vi "CreateItemsString.vi"(11 "Items":string[](array[string])=["C1", "C2", "C3"]) -> (1 "Items for SELECT":string, 2 "Items for INSERT":string, 3 "Items for CREATE":string)   [LabVIEW 2015, in "DBToolkit.lvlib"]
uses:
  DBToolkit.lvlib
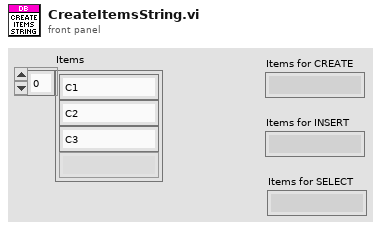
[diagram p1: front panel]
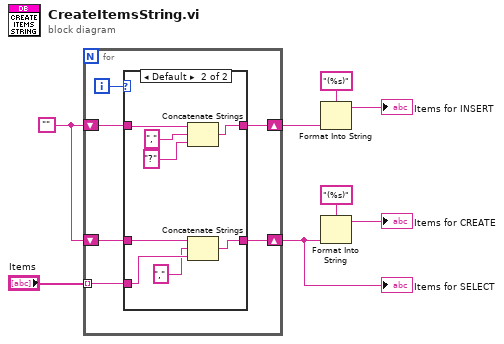
[diagram p0: block diagram]
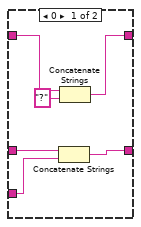
[diagram p2: hidden frame]
diagram:
  w7 = ""
  n1 = for {
    shift-right: [w11] -> w1
    shift-left: w7 -> [w13]
    tunnel: "Items" -> [w12] mode=indexing
    shift-right: [w9] -> w5
    shift-left: w7 -> [w10]
    i -> [w14]
    n2 = case shown="Default" w14 {
      tunnel: w13 -> [w20 w26]
      tunnel: w12 -> [w19 w28]
      tunnel: [w18 w27] -> w11
      tunnel: w10 -> [w17 w22]
      tunnel: [w15 w23] -> w9
      frame 0 {
        n3 = Concatenate Strings(w20, w19) -> (w18:string)
        n4 = Concatenate Strings(w17, "?" ("string")) -> (w15:string)
      }
      frame Default {
        n5 = Concatenate Strings(w22, ",", "?" ("string")) -> (w23:string)
        n6 = Concatenate Strings(w26, ",", w28) -> (w27:string)
      }
    }
  }
  "Items for SELECT" <- w1
  n7 = Format Into String(format string="(%s)", w5) -> (resulting string=→"Items for INSERT":string)  [unwired: 2 in, 1 out]
  n8 = Format Into String(format string="(%s)", w1) -> (resulting string=→"Items for CREATE":string)  [unwired: 2 in, 1 out]
